vi "XIPIN_32-bit_Initiator_Target_for_PCI_(7-Series)_5_0.vi"   [LabVIEW 2017]
doc: "With the Xilinx LogiCORE 32-bit Initiator/Target v4 for PCI, a designer can build a customized PCI 3.0 compliant design with performance approaching 266 Mbytes/sec. PCI is a popular bus standard, not only for personal computers, but also for industrial computers, communication switches, routers and instrumentation.\n------------------------------------\n<b>Need License</b> : Yes"
uses:
  <vilib>/rvi/XilinxIP/XIPIN_XNode/niFpgaXIPIN.xnode
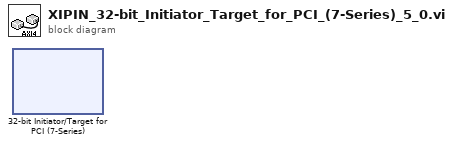
[diagram p0: block diagram]
diagram:
  n1 = xnode ("32-bit Initiator/Target for PCI (7-Series)")() -> ()
